vi "LabVLC - PlayControl.vi"(2 "error in (no error)":errorcluster, 3 "struct":T1={"media_ptr"=0, "vlc_inst_ptr"=0, "path in"=path "C:/Program Files (x86)/VideoLAN/VLC/libvlc.dll"}) -> (0 "error out":errorcluster, 1 "output cluster":T1)   [LabVIEW 2014]
doc: "Play the video in the VLC player. May be called anytime after initialization. Requires a media pointer. The ramifications of calling stop or pause before this function are unknown."
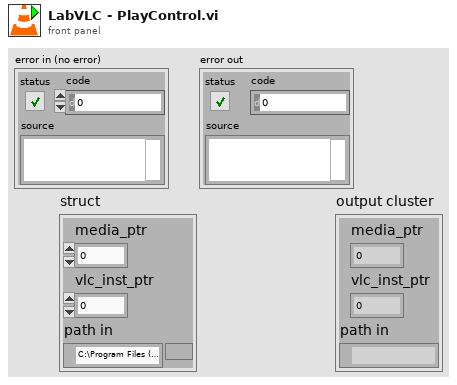
[diagram p1: front panel]
types:
  T1 = cluster{"media_ptr":i32, "vlc_inst_ptr":i32, "path in":path}
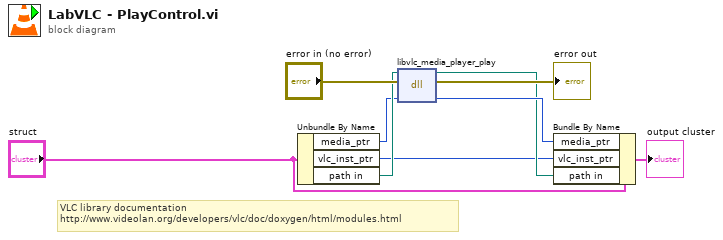
[diagram p0: block diagram]
diagram:
  # "VLC library documentation\nhttp://www.videolan.org/developers/vlc/doc/doxygen/html/modules.html"
  n1 = Unbundle By Name("struct") -> ("media_ptr"=w6:i32, "vlc_inst_ptr"=w1:i32, "path in"=w7:path)
  n2 = dll-call lib="C:/Program Files (x86)/VideoLAN/VLC/libvlc.dll" fn="libvlc_media_player_play"(path in=w7, error in="error in (no error)", "p_mi"=w6) -> (path out=w4:path, error out=→"error out":errorcluster, "p_mi"=w5:i32)  [unwired: 2 in]
  n3 = Bundle By Name(cluster="struct", "media_ptr"=w5, "vlc_inst_ptr"=w1, "path in"=w4) -> (→"output cluster":T1)
